vi "Untitled 4.vi"() -> ()   [LabVIEW 2011]
panel:
  in  "stepsize::1":dbl=0.02 caption="stepsize" min=0.0 max=10.0
  in  "vangle::1 3":dbl caption="v" min=-5.0 max=5.0
  in  "ypos::1 3":dbl=4.0 caption="y" min=-20.0 max=20.0
  in  "vangle::1 2":dbl caption="v" min=-5.0 max=5.0
  in  "ypos::1 2":dbl=4.0 caption="y" min=-20.0 max=20.0
  in  "vangle::1":dbl caption="v" min=-5.0 max=5.0
  in  "ypos::1":dbl=4.0 caption="y" min=-20.0 max=20.0
  in  "relativemove.ypos::7":bool
  in  "relativemove.xpos::7":bool
  in  "relativemove.yneg::7":bool
  in  "relativemove.xneg::7":bool
  in  "relativemove.zpos::7":bool
  in  "relativemove.zneg::7":bool
  in  "relativemove.wpos::7":bool
  in  "relativemove.upos::7":bool
  in  "relativemove.uneg::7":bool
  in  "relativemove.vpos::7":bool
  in  "relativemove.vneg::7":bool
  in  "relativemove.wneg::7":bool
  # "Z"
  # "+"
  # "Y"
  # "+"
  # "-"
  # "+"
  # "-"
  # "-"
  # "X"
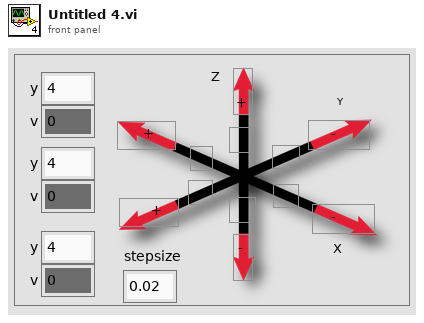
[diagram p1: front panel]
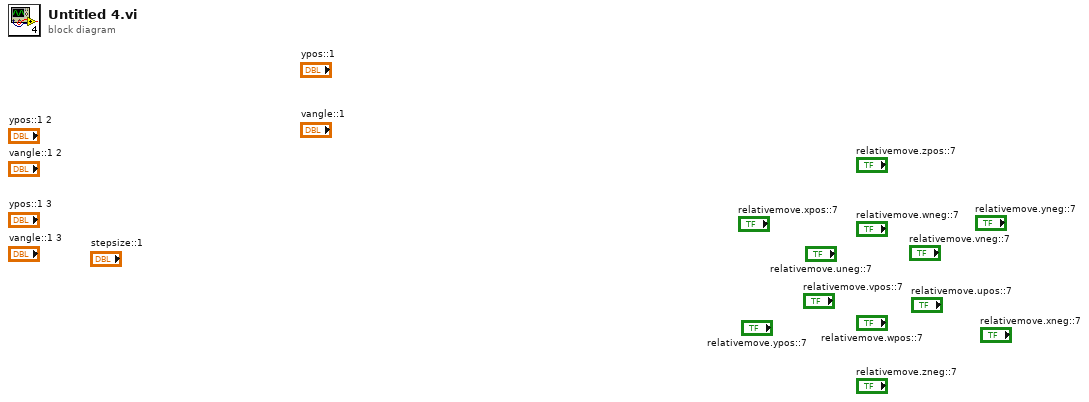
[diagram p0: block diagram]
diagram:
